vi "Action.vi"(8 "error in (no error)":errorcluster, 10 "OOQMH in":refnum<class "OOQMH.lvclass">, 11 "Set PID Gains in":refnum<class "Set PID Gains.lvclass">) -> (0 "error out":errorcluster, 2 "OOQMH out":refnum<class "OOQMH.lvclass">, 3 "Set PID Gains out":refnum<class "Set PID Gains.lvclass">)   [LabVIEW 2024, in "PID Loop.lvlib" / "Set PID Gains.lvclass"]
uses:
  OOQMH/OOQMH/OOQMH.lvclass
  Set PID Gains.lvclass
  Set PID Gains.lvclass/Set PID Gains.ctl
  PID Loop/PID Loop.lvclass
  C:/Users/uspoaotto/OneDrive - Oregon Tool/Desktop/working copies/helperLoop/src/OOQMH/OOQMH/OOQMH.lvclass
  C:/Users/uspoaotto/OneDrive - Oregon Tool/Desktop/working copies/helperLoop/src/PID Loop/PID Loop/PID Loop.lvclass
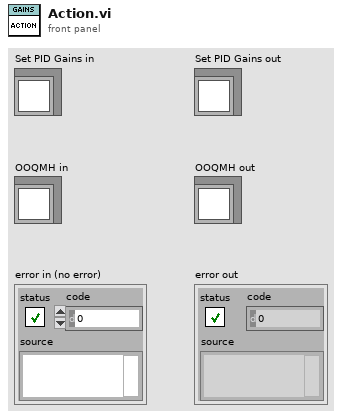
[diagram p1: front panel]
types:
  T1 = cluster{"proportional gain (Kc)":dbl, "integral time (Ti, min)":dbl, "derivative time (Td, min)":dbl}
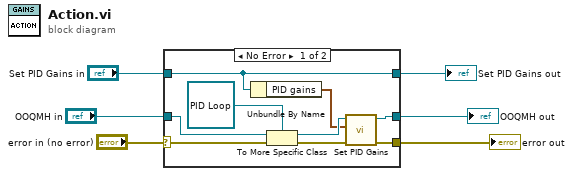
[diagram p0: block diagram]
diagram:
  n1 = case shown="No Error" "error in (no error)" {
    selector: "error in (no error)" -> [w12 w18]
    tunnel: [w15 w18] -> w5
    tunnel: "OOQMH in" -> [w13 w17]
    tunnel: [w9 w17] -> w3
    tunnel: [w8 w16] -> w2
    tunnel: "Set PID Gains in" -> [w8 w16]
    frame No Error {
      n2 = Unbundle By Name(w8) -> ("PID gains"=w7:T1)
      n3 = To More Specific Class(target class=refnum<class "PID Loop.lvclass"> refnum ("PID Loop in"), reference=w13, error in=w12) -> (specific class reference=w10:refnum<class "PID Loop.lvclass">, error out=w11:errorcluster)
      n4 = call-dynamic "Set PID Gains.vi"("error in (no error)"=w11, "PID gains"=w7, "PID Loop in"=w10) -> ("error out"=w15:errorcluster, "PID Loop out"=w9:refnum<class "PID Loop.lvclass">)  [unwired: 7 in]
    }
    frame Error {
    }
  }
  "error out" <- w5
  "Set PID Gains out" <- w2
  "OOQMH out" <- w3
